vi "WSVCAP SHL Host TL Close.vi"(11 "error in":errorcluster, 14 "FPGA":T1) -> (15 "error out":errorcluster)   [LabVIEW 2017]
uses:
  Type Defs/WSVCAP SHL FPGA Enum.ctl
  Type Defs/WSVCAP SHL Function Enum.ctl
  Type Defs/WSVCAP SHL Gatekeeper Operation Enum.ctl
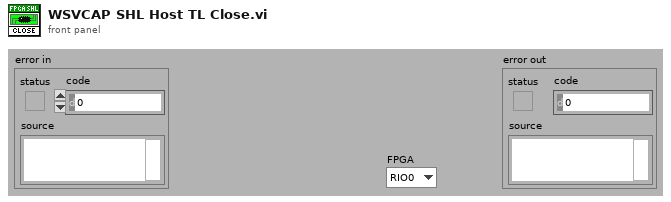
[diagram p1: front panel]
types:
  T1 = typedef "WSVCAP SHL FPGA Enum.ctl" = enum16{"RIO0", "RIO1"}
  T2 = typedef "WSVCAP SHL Gatekeeper Operation Enum.ctl" = enum16{"Initialize", "Lock", "Unlock", "Close"}
  T3 = typedef "WSVCAP SHL Function Enum.ctl" = enum16{"Initialize", "Configure I2C", "Configure SRL", "Write I2C", "Read I2C", "Write SRL", "Start SRL Cycle", "Stop SRL Cycle", "Get Status", "Close"}
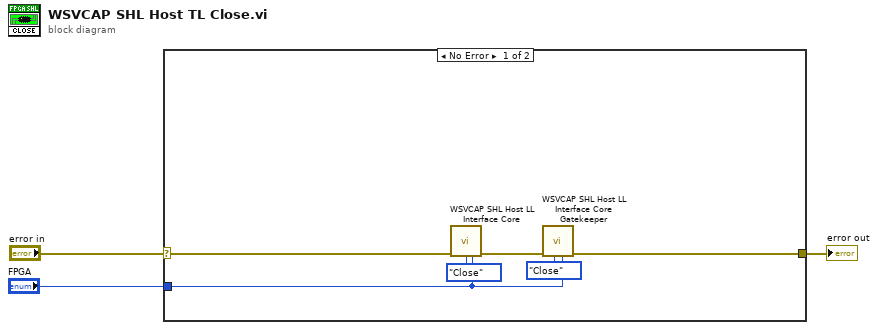
[diagram p0: block diagram]
diagram:
  n1 = case shown="No Error" "error in" {
    selector: "error in" -> [w9 w10]
    tunnel: [w5 w10] -> w2
    tunnel: "FPGA" -> [w4 _]
    frame No Error {
      n2 = call "WSVCAP SHL Host LL Interface Core.vi"("error in"=w9, "Function"=WSVCAP_SHL_Function_Enum."Close", "FPGA"=w4) -> ("error out"=w6:errorcluster)  [unwired: 10 in, 2 out]
      n3 = call "WSVCAP SHL Host LL Interface Core Gatekeeper.vi"("FPGA"=w4, "Operation"=WSVCAP_SHL_Gatekeeper_Operation_Enum."Close", "error in (no error)"=w6) -> ("error out"=w5:errorcluster)  [unwired: 8 in]
    }
    frame Error {
    }
  }
  "error out" <- w2
